vi "Raw Values Reading.vi"() -> ()   [LabVIEW 2014]
uses:
  <vilib>/Aledyne-TSXperts/Arduino Compatible Compiler for LabVIEW/Code Generator/Arduino APIs/I2C/I2C Mode.ctl
  <vilib>/Aledyne-TSXperts/Arduino Compatible Compiler for LabVIEW/Code Generator/Arduino APIs/I2C/I2C Write Array.vi
  <vilib>/Aledyne-TSXperts/Arduino Compatible Compiler for LabVIEW/Arduino Compatible Compiler for LabVIEW.lvlib
  <vilib>/Aledyne-TSXperts/Arduino Compatible Compiler for LabVIEW/addons/Arduino MPU60X0/Arduino MPU60X0.lvlib
panel:
  out "error out":errorcluster
  in  "error in (no error)":errorcluster
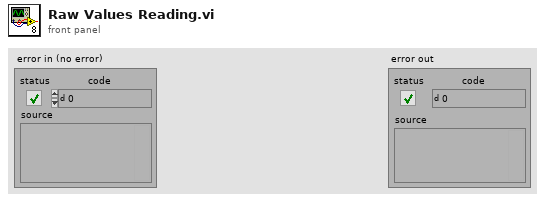
[diagram p1: front panel]
types:
  T1 = typedef "Arduino Compatible Compiler for LabVIEW.lvlib/I2C Mode.ctl" = enum16{"Master", "Slave"}
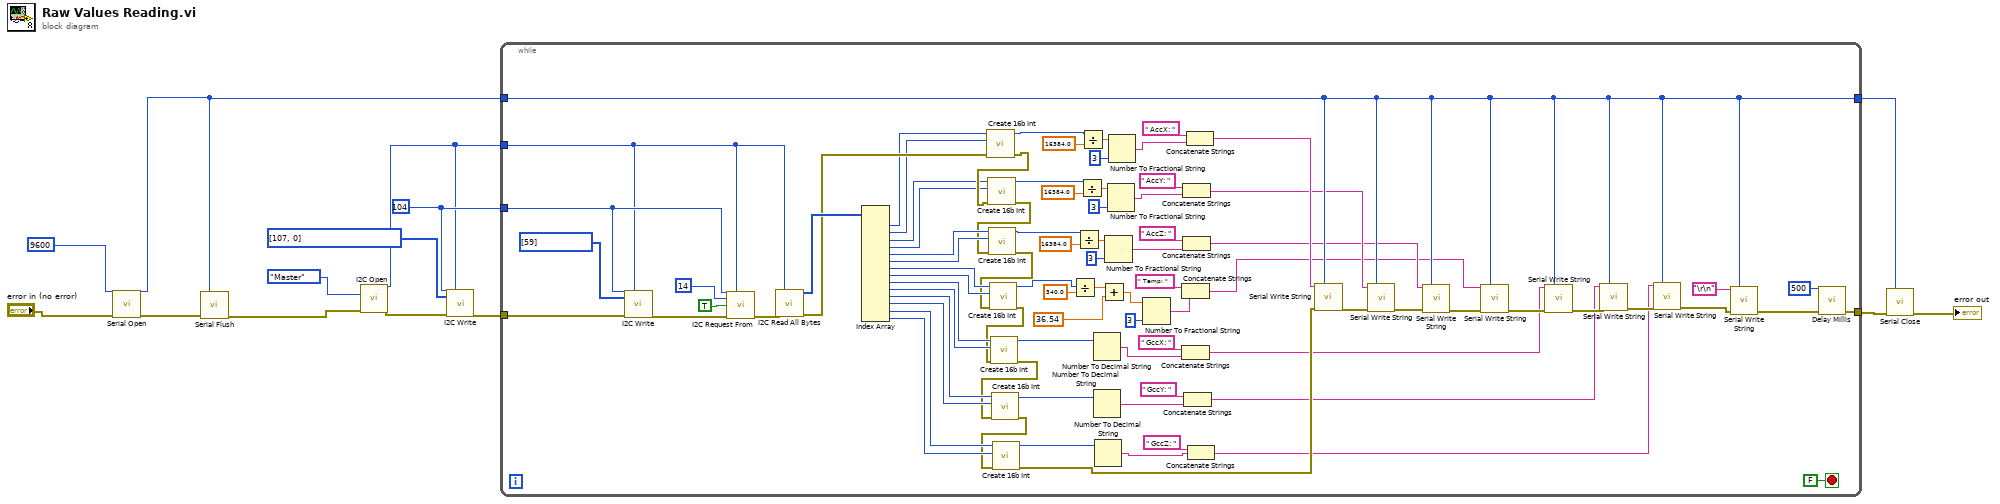
[diagram p0: block diagram]
diagram:
  w11 = u8 104 ("Slave Address")
  n1 = call <vilib>:"Serial Open.vi"("Speed"=u32 9600, "error in (no error)"="error in (no error)") -> ("Instance"=w3:u8, "error out"=w5:errorcluster)  [unwired: 12 in]
  n2 = call <vilib>:"Serial Flush.vi"("Instance"=w3, "error in (no error)"=w5) -> ("error out"=w6:errorcluster)  [unwired: 13 in]
  n3 = call <vilib>:"I2C Open.vi"("Mode"=I2C_Mode."Master", "error in (no error)"=w6) -> ("Interface"=w9:u8, "error out"=w13:errorcluster)  [unwired: 12 in]
  n4 = call-poly <vilib>:"I2C Write.vi"("Slave Address"=w11, "Interface"=w9, "Data"=u8[] [107, 0], "error in (no error)"=w13) -> ("error out"=w10:errorcluster)  [unwired: 10 in, 1 out]
  n5 = while {
    tunnel: w11 -> [w98]
    tunnel: w10 -> [w95]
    tunnel: w9 -> [w88]
    tunnel: [w93] -> w8
    tunnel: w3 -> [w55]
    tunnel: [w55] -> w2
    stop <- FALSE stop-if-true
    n6 = call-poly <vilib>:"I2C Write.vi"("Slave Address"=w98, "Interface"=w88, "Data"=u8[] [59], "error in (no error)"=w95) -> ("error out"=w99:errorcluster)  [unwired: 10 in, 1 out]
    n7 = call <vilib>:"I2C Request From.vi"("Slave Address"=w98, "Interface"=w88, "Number of Bytes"=u32 14, "Send Stop"=TRUE, "error in (no error)"=w99) -> ("error out"=w89:errorcluster)  [unwired: 10 in]
    n8 = call <vilib>:"I2C Read All Bytes.vi"("Interface"=w88, "error in (no error)"=w89) -> ("Data"=w87:u8[], "error out"=w76:errorcluster)  [unwired: 12 in]
    n9 = Index Array(array=w87) -> (element #1=w40:u8, element #2=w39:u8, element #3=w38:u8, element #4=w37:u8, element #5=w86:u8, element #6=w85:u8, element #7=w84:u8, element #8=w83:u8, element #9=w82:u8, element #10=w81:u8, element #11=w80:u8, element #12=w79:u8, element #13=w78:u8, element #14=w77:u8)  [unwired: 14 in]
    n10 = call <vilib>:"Create 16b Int.vi"("Error In"=w76, "LSB"=w39, "MSB"=w40) -> ("Error Out"=w75:errorcluster, "Int"=w35:i16)  [unwired: 7 in]
    n11 = call <vilib>:"Create 16b Int.vi"("Error In"=w75, "LSB"=w37, "MSB"=w38) -> ("Error Out"=w74:errorcluster, "Int"=w28:i16)  [unwired: 7 in]
    n12 = call <vilib>:"Create 16b Int.vi"("Error In"=w74, "LSB"=w85, "MSB"=w86) -> ("Error Out"=w73:errorcluster, "Int"=w24:i16)  [unwired: 7 in]
    n13 = call <vilib>:"Create 16b Int.vi"("Error In"=w73, "LSB"=w83, "MSB"=w84) -> ("Error Out"=w72:errorcluster, "Int"=w18:i16)  [unwired: 7 in]
    n14 = call <vilib>:"Create 16b Int.vi"("Error In"=w72, "LSB"=w81, "MSB"=w82) -> ("Error Out"=w71:errorcluster, "Int"=w69:i16)  [unwired: 7 in]
    n15 = call <vilib>:"Create 16b Int.vi"("Error In"=w71, "LSB"=w79, "MSB"=w80) -> ("Error Out"=w70:errorcluster, "Int"=w68:i16)  [unwired: 7 in]
    n16 = call <vilib>:"Create 16b Int.vi"("Error In"=w70, "LSB"=w77, "MSB"=w78) -> ("Error Out"=w56:errorcluster, "Int"=w67:i16)  [unwired: 7 in]
    n17 = Divide(x=w18, y=340.0) -> (x/y=w17:dbl)
    n18 = Divide(x=w24, y=16384.0) -> (x/y=w26:dbl)
    n19 = Divide(x=w28, y=16384.0) -> (x/y=w30:dbl)
    n20 = Divide(x=w35, y=16384.0) -> (x/y=w34:dbl)
    n21 = Number To Decimal String(number=w69) -> (decimal integer string=w59:string)  [unwired: 1 in]
    n22 = Number To Decimal String(number=w68) -> (decimal integer string=w58:string)  [unwired: 1 in]
    n23 = Number To Decimal String(number=w67) -> (decimal integer string=w57:string)  [unwired: 1 in]
    n24 = Add(x=w17, y=36.54) -> (x+y=w15:dbl)
    n25 = Number To Fractional String(number=w26, precision (6)=i16 3) -> (F-format string=w23:string)  [unwired: 2 in]
    n26 = Number To Fractional String(number=w30, precision (6)=i16 3) -> (F-format string=w22:string)  [unwired: 2 in]
    n27 = Number To Fractional String(number=w34, precision (6)=i16 3) -> (F-format string=w33:string)  [unwired: 2 in]
    n28 = Number To Fractional String(number=w15, precision (6)=i16 3) -> (F-format string=w19:string)  [unwired: 2 in]
    n29 = Concatenate Strings(" Temp: " ("string"), w19) -> (w45:string)
    n30 = Concatenate Strings(" GccX: " ("string"), w59) -> (w44:string)
    n31 = Concatenate Strings(" AccY: " ("string"), w22) -> (w47:string)
    n32 = Concatenate Strings(" AccZ: " ("string"), w23) -> (w46:string)
    n33 = Concatenate Strings(" GccY: " ("string"), w58) -> (w43:string)
    n34 = Concatenate Strings(" AccX: " ("string"), w33) -> (w48:string)
    n35 = Concatenate Strings(" GccZ: " ("string"), w57) -> (w42:string)
    n36 = call <vilib>:"Serial Write String.vi"("String"=w48, "Instance"=w55, "error in (no error)"=w56) -> ("error out"=w54:errorcluster)  [unwired: 12 in]
    n37 = call <vilib>:"Serial Write String.vi"("String"=w47, "Instance"=w55, "error in (no error)"=w54) -> ("error out"=w53:errorcluster)  [unwired: 12 in]
    n38 = call <vilib>:"Serial Write String.vi"("String"=w46, "Instance"=w55, "error in (no error)"=w53) -> ("error out"=w52:errorcluster)  [unwired: 12 in]
    n39 = call <vilib>:"Serial Write String.vi"("String"=w45, "Instance"=w55, "error in (no error)"=w52) -> ("error out"=w51:errorcluster)  [unwired: 12 in]
    n40 = call <vilib>:"Serial Write String.vi"("String"=w44, "Instance"=w55, "error in (no error)"=w51) -> ("error out"=w50:errorcluster)  [unwired: 12 in]
    n41 = call <vilib>:"Serial Write String.vi"("String"=w43, "Instance"=w55, "error in (no error)"=w50) -> ("error out"=w49:errorcluster)  [unwired: 12 in]
    n42 = call <vilib>:"Serial Write String.vi"("String"=w42, "Instance"=w55, "error in (no error)"=w49) -> ("error out"=w41:errorcluster)  [unwired: 12 in]
    n43 = call <vilib>:"Serial Write String.vi"("String"="\r\n" ("End of Line Constant"), "Instance"=w55, "error in (no error)"=w41) -> ("error out"=w91:errorcluster)  [unwired: 12 in]
    n44 = call <vilib>:"Delay Millis.vi"("error in (no error)"=w91, "delay"=u32 500) -> ("error out"=w93:errorcluster)  [unwired: 9 in]
  }
  n45 = call <vilib>:"Serial Close.vi"("Instance"=w2, "error in (no error)"=w8) -> ("error out"=→"error out":errorcluster)  [unwired: 13 in]
